vi "LV8_1.vi"() -> ()   [LabVIEW 2011]
uses:
  <vilib>/Analysis/1siggen.llb/Ramp Pattern by Samples.vi
  <vilib>/Analysis/NI_AALBase.lvlib
panel:
  in  "Pole/Zero Location (r/theta) 6":T1={"r"=0.8, "q (in p)"=0.5, "pz"=TRUE, "enable\nenable"=TRUE} {"q (in p)" min=0.0 max=1.0 step=0.1; "r" min=0.0 step=0.1}
  in  "Pole/Zero Location (r/theta) 5":T2={"r"=0.8, "q (in p)"=0.25, "pz"=TRUE, "enable"=TRUE} {"q (in p)" min=0.0 max=1.0 step=0.1; "r" min=0.0 step=0.1}
  in  "Pole/Zero Location (r/theta) 4":T2={"r"=0.6, "q (in p)"=0.0, "pz"=TRUE, "enable"=TRUE} {"q (in p)" min=0.0 max=1.0 step=0.1; "r" min=0.0 step=0.1}
  in  "Pole/Zero Location (r/theta) 3":T2={"r"=1.0, "q (in p)"=1.0, "pz"=FALSE, "enable"=TRUE} {"q (in p)" min=0.0 max=1.0 step=0.1; "r" min=0.0 step=0.1}
  in  "Pole/Zero Location (r/theta) 2":T2={"r"=1.0, "q (in p)"=0.75, "pz"=FALSE, "enable"=TRUE} {"q (in p)" min=0.0 max=1.0 step=0.1; "r" min=0.0 step=0.1}
  out "Y":dbl=1.4000000000000004 min=0.0 max=1.2000000000000002 step=0.1 format="%.3g"
  in  "X":dbl min=0.0 max=3.15 step=0.1 format="%.3g"
  in  "Max FR Mag":dbl=1.4000000000000004 min=1e-05 step=0.1 format="%.3g"
  in  "stop":bool
  out "Gain K":dbl=0.03420443704820256 format="%#.3g"
  out "Pole-Zero Plot":cluster{"Y":dbl[], "Y":dbl[]}[](graph)=[{"Y"=array[4001 elements], "Y"=array[4001 elements]}, {"Y"=[0.6, 0.6, 0.565685424949238, 0.565685424949238, 4.898425415289509e-17, 4.898425415289509e-17], "Y"=[0.0, -0.0, 0.565685424949238, -0.565685424949238, 0.8, -0.8]}, {"Y"=[6.123031769111886e-17, 6.123031769111886e-17, -0.7071067811865475, -0.7071067811865475, -1.0, -1.0], "Y"=[1.0, -1.0, 0.7071067811865476, -0.7071067811865476, 1.2246063538223773e-16, -1.2246063538223773e-16]}, {"Y"=[0.0, 1.0], "Y"=[0.0, 0.0]}]
  out "Magnitude of Frequency Response":cluster{dbl[], "Ramp Pattern":dbl[]}(graph)
  in  "Pole/Zero Location (r/theta) 1":T2={"r"=1.0, "q (in p)"=0.5, "pz"=FALSE, "enable"=TRUE} {"q (in p)" min=0.0 max=1.0 step=0.1; "r" min=0.0 step=0.1}
  # "Filter Design by Pole-Zero Placement"
  # "Vertical Cursor"
  # "+/-"
  # "+/-"
  # "+/-"
  # "+/-"
  # "+/-"
  # "+/-"
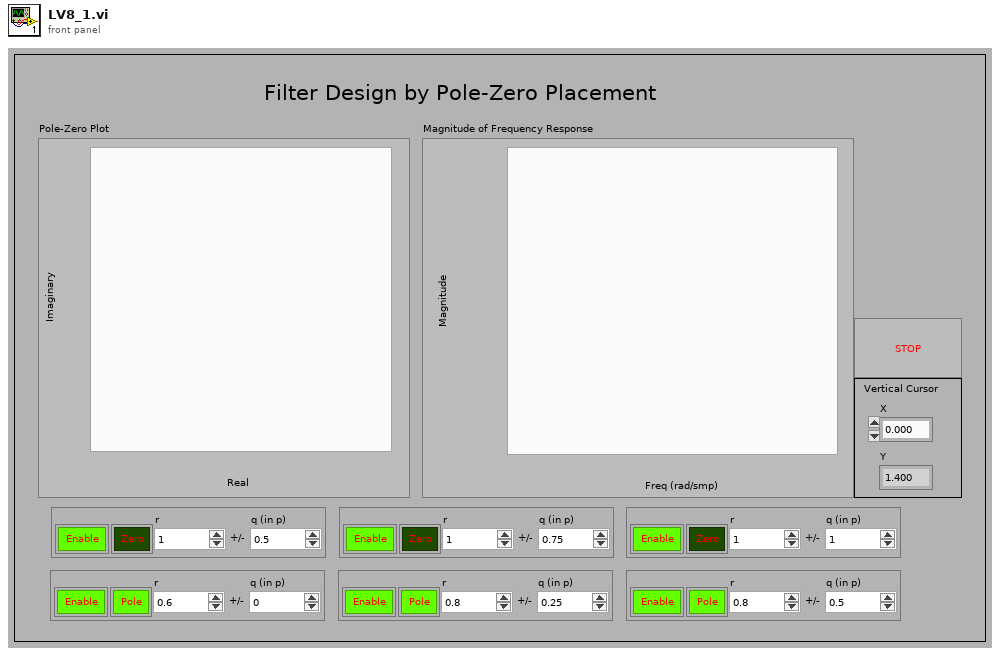
[diagram p1: front panel]
types:
  T1 = cluster{"r":dbl, "q (in p)":dbl, "pz":bool, "enable\nenable":bool}
  T2 = cluster{"r":dbl, "q (in p)":dbl, "pz":bool, "enable":bool}
  T3 = cluster{"r":dbl, "q (in p)":dbl, "pz":bool, "enable\nenable":bool}[]
  T4 = typedef "LVPointDoubleTypeDef.ctl" = cluster{"Cursor X":dbl, "Cursor Y":dbl}
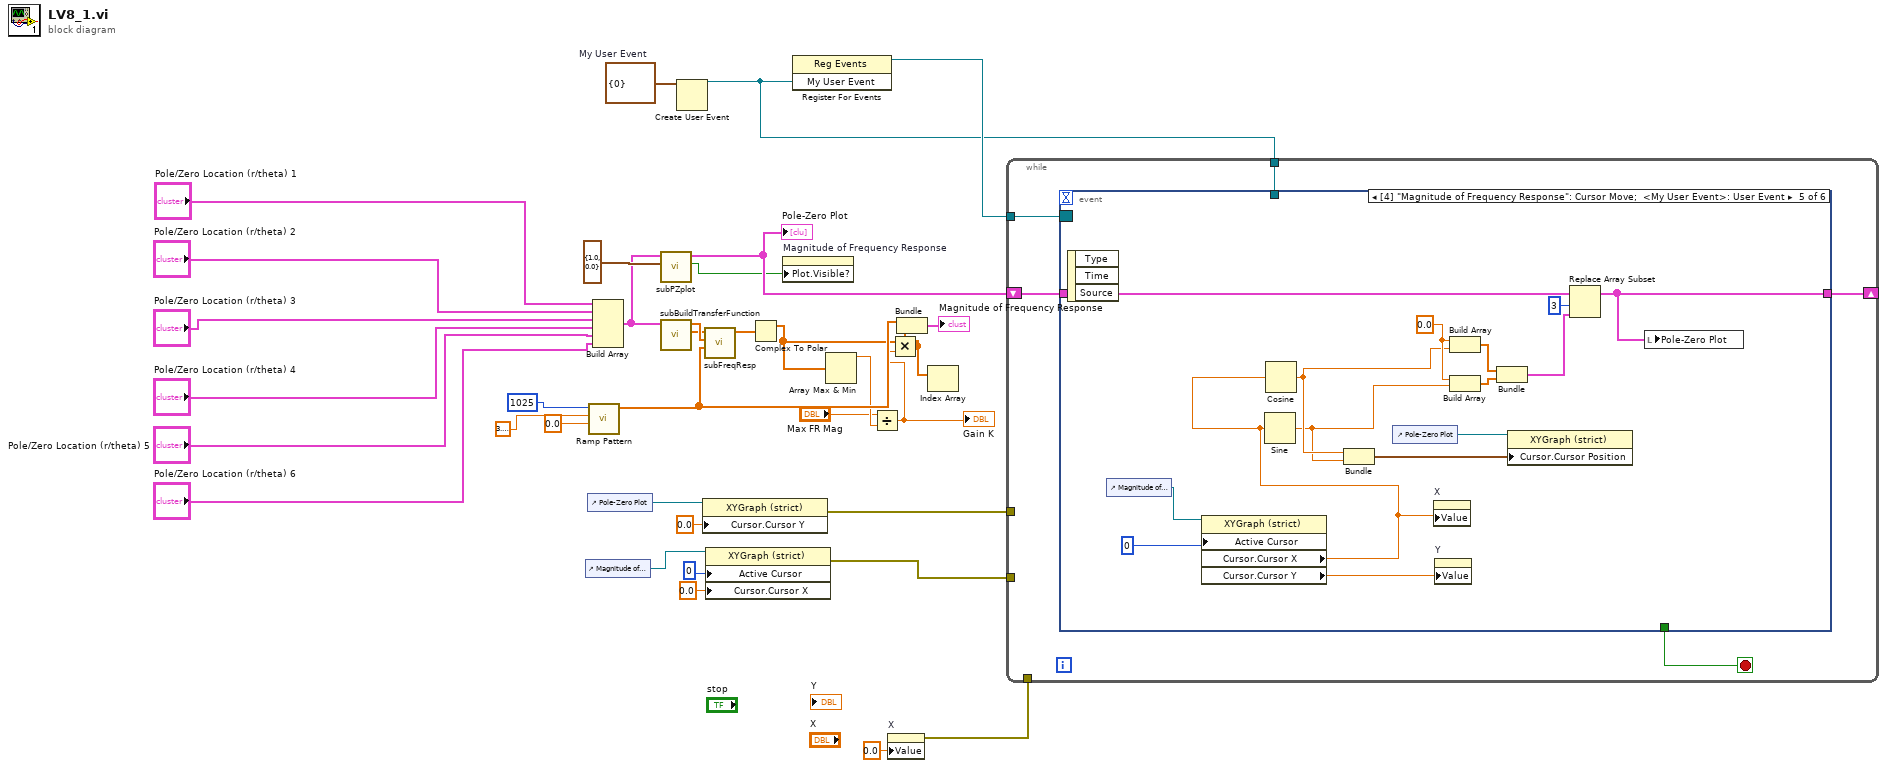
[diagram p0: block diagram]
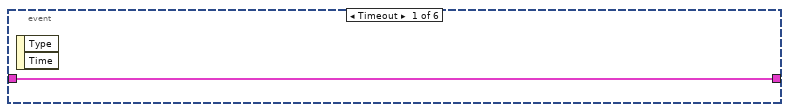
[diagram p2: hidden frame]
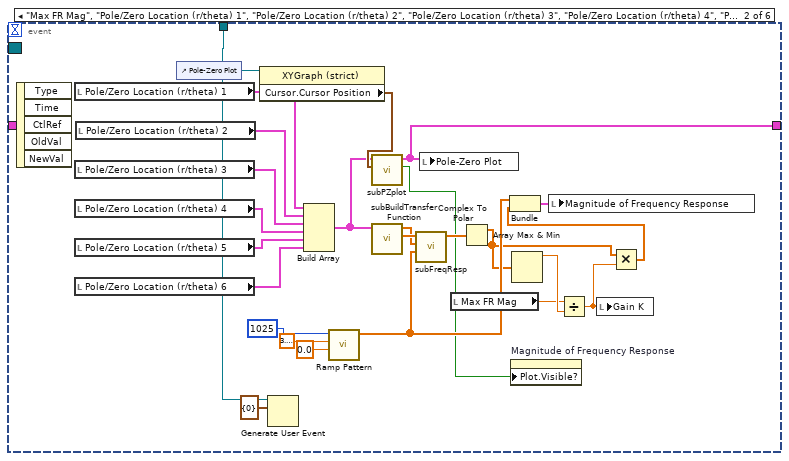
[diagram p3: hidden frame]
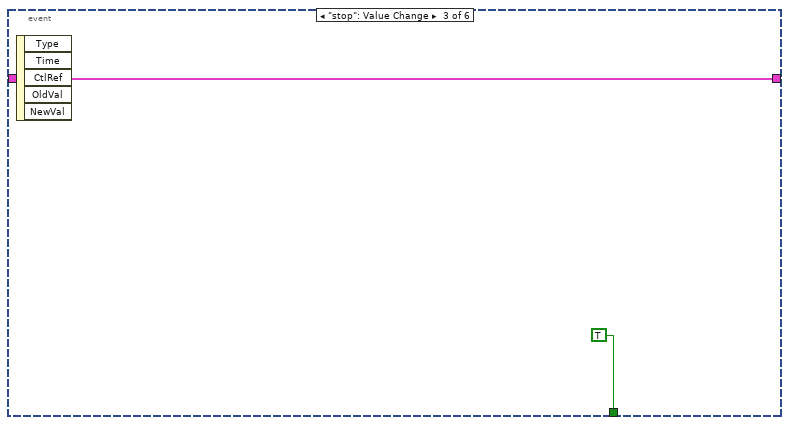
[diagram p4: hidden frame]
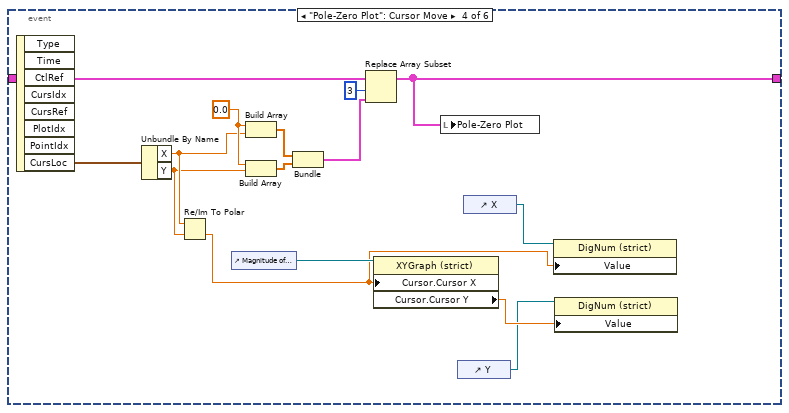
[diagram p5: hidden frame]
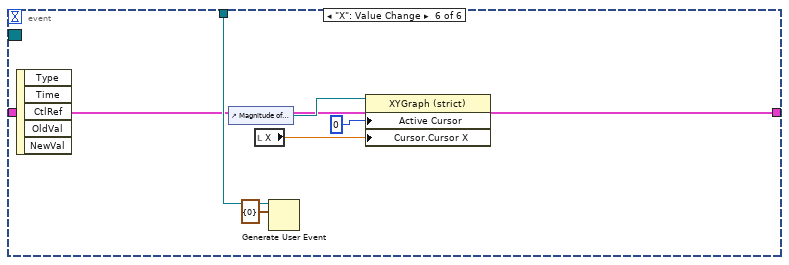
[diagram p6: hidden frame]
diagram:
  w16 = cluster{"dummy":i32} {"dummy"=0}  # My User Event
  n1 = control-ref of="Magnitude of Frequency Response"() -> (w22:refnum<vi>)
  n2 = control-ref of="Pole-Zero Plot"() -> (w25:refnum<vi>)
  n3 = call-poly <vilib>:"Ramp Pattern.vi"("start"=0.0, "end"=3.141592653589793, "samples"=1025) -> ("Ramp Pattern"=w32:dbl[])  [unwired: 7 in, 1 out]
  n4 = Build Array("Pole/Zero Location (r/theta) 1", "Pole/Zero Location (r/theta) 2", "Pole/Zero Location (r/theta) 3", "Pole/Zero Location (r/theta) 4", "Pole/Zero Location (r/theta) 5", "Pole/Zero Location (r/theta) 6") -> (w2:T3)
  n5 = call "subPZplot.vi"("cursor pos"=cluster{"x":dbl, "y":dbl} {"x"=1.0, "y"=0.0}, "PZarray"=w2) -> ("stable？"=w19:bool, "PZplot"=w29:cluster{"Y":dbl[], "Y":dbl[]}[])  [unwired: 8 in]
  "Pole-Zero Plot" <- w29
  n6 = call "subBuildTransferFunction.vi"("PZarray"=w2) -> ("a"=w27:dbl[], "b"=w26:dbl[])  [unwired: 8 in]
  n7 = Create User Event(user event datatype=w16) -> (user event=w15:refnum<user-event>)  [unwired: 1 in, 1 out]
  n8 = property class="XYGraph (strict)"(reference=w25, "Cursor.Cursor Y"=0.0 ("Cursor.Cursor Position:Cursor Y")) -> (error out=w23:errorcluster)  [unwired: 1 in, 1 out]
  n9 = call "subFreqResp.vi"("omega"=w32, "a"=w27, "b"=w26) -> ("Frequency Response"=w35:cdb[])  [unwired: 8 in]
  n10 = property class="XYGraph (strict)"(reference=w22, "Active Cursor"=u32 0, "Cursor.Cursor X"=0.0 ("Cursor.Cursor Position:Cursor Y")) -> (error out=w21:errorcluster)  [unwired: 1 in, 1 out]
  n11 = Complex To Polar(r * e^(i*theta)=w35) -> (r=w13:dbl[])  [unwired: 1 out]
  n12 = property on="Magnitude of Frequency Response" class="XYGraph (strict)"("Plot.Visible?"=w19) -> ()  [unwired: 2 in, 2 out]
  n13 = register-events(w15) -> (reference out=w17:refnum<event-registration>)  [unwired: 2 in, 1 out]
  n14 = Array Max & Min(array=w13) -> (max value=w18:dbl)  [unwired: 3 out]
  n15 = Divide(x="Max FR Mag", y=w18) -> (x/y=w12:dbl)
  "Gain K" <- w12
  n16 = property on="X" class="DigNum (strict)"("Value"=0.0 ("X")) -> (error out=w1:errorcluster)  [unwired: 2 in, 1 out]
  n17 = Multiply(x=w13, y=w12) -> (x*y=w11:dbl[])
  n18 = Bundle("Ramp Pattern"=w32, w11) -> (→"Magnitude of Frequency Response":cluster{"Ramp Pattern":dbl[], dbl[]})  [unwired: 1 in]
  n19 = Index Array(array=w11) -> ()  [unwired: 1 in, 1 out]
  n20 = while {
    shift-right: [w39] -> _
    shift-left: w29 -> [w40]
    tunnel: w23 -> [_]
    tunnel: w21 -> [_]
    tunnel: w17 -> [w37]
    tunnel: w15 -> [w36]
    tunnel: w1 -> [_]
    stop <- w38 stop-if-true
    n21 = event shown="[4] \"Magnitude of Frequency Response\": Cursor Move;  <My User Event>: User Event" {
      selector: w37 -> [_ _ _ _ _ _]
      dyn-events: _ -> [_ _ _ _ _ _]
      timeout: _ -> [_ _ _ _ _ _]
      tunnel: w40 -> [w41 _ w68 w80 w94 w101]
      tunnel: [w41 w58 _ w77 w93 w101] -> w39
      tunnel: [_ _ TRUE _ _ _] -> w38
      tunnel: [_ _ w68 _ _ _] -> _
      tunnel: w36 -> [_ w50 _ _ _ w104]
      event Timeout {
        n22 = event-data() -> ()  [unwired: 1 in, 2 out]
      }
      event "Max FR Mag", "Pole/Zero Location (r/theta) 1", "Pole/Zero Location (r/theta) 2", "Pole/Zero Location (r/theta) 3", "Pole/Zero Location (r/theta) 4", "Pole/Zero Location (r/theta) 5", "Pole/Zero Location (r/theta) 6": Value Change {
        n23 = event-data() -> ()  [unwired: 1 in, 5 out]
        n24 = local read "Pole/Zero Location (r/theta) 1"() -> (w65:T2)
        n25 = local read "Pole/Zero Location (r/theta) 3"() -> (w46:T2)
        n26 = local read "Pole/Zero Location (r/theta) 4"() -> (w45:T2)
        n27 = local read "Pole/Zero Location (r/theta) 5"() -> (w44:T2)
        n28 = local read "Pole/Zero Location (r/theta) 6"() -> (w43:T1)
        n29 = local read "Pole/Zero Location (r/theta) 2"() -> (w47:T2)
        n30 = control-ref of="Pole-Zero Plot"() -> (w67:refnum<vi>)
        n31 = property class="XYGraph (strict)"(reference=w67) -> ("Cursor.Cursor Position"=w57:T4)  [unwired: 1 in, 2 out]
        n32 = Generate User Event(user event=w50, event data cluster=cluster{"dummy":i32} {"dummy"=0} ("event data")) -> ()  [unwired: 1 in, 2 out]
        n33 = Build Array(w65, w47, w46, w45, w44, w43) -> (w42:T3)
        n34 = call-poly <vilib>:"Ramp Pattern.vi"("start"=0.0, "end"=3.141592653589793, "samples"=1025) -> ("Ramp Pattern"=w59:dbl[])  [unwired: 7 in, 1 out]
        n35 = call "subPZplot.vi"("cursor pos"=w57, "PZarray"=w42) -> ("stable？"=w55:bool, "PZplot"=w58:cluster{"Y":dbl[], "Y":dbl[]}[])  [unwired: 8 in]
        n36 = call "subBuildTransferFunction.vi"("PZarray"=w42) -> ("a"=w63:dbl[], "b"=w64:dbl[])  [unwired: 8 in]
        n37 = call "subFreqResp.vi"("omega"=w59, "a"=w63, "b"=w64) -> ("Frequency Response"=w60:cdb[])  [unwired: 8 in]
        n38 = local write "Pole-Zero Plot"(w58) -> ()
        n39 = local read "Max FR Mag"() -> (w48:dbl)
        n40 = Complex To Polar(r * e^(i*theta)=w60) -> (r=w53:dbl[])  [unwired: 1 out]
        n41 = property on="Magnitude of Frequency Response" class="XYGraph (strict)"("Plot.Visible?"=w55) -> ()  [unwired: 2 in, 2 out]
        n42 = Array Max & Min(array=w53) -> (max value=w54:dbl)  [unwired: 3 out]
        n43 = Divide(x=w48, y=w54) -> (x/y=w52:dbl)
        n44 = local write "Gain K"(w52) -> ()
        n45 = Multiply(x=w53, y=w52) -> (x*y=w51:dbl[])
        n46 = Bundle("Ramp Pattern"=w59, w51) -> (w66:cluster{"Ramp Pattern":dbl[], dbl[]})  [unwired: 1 in]
        n47 = local write "Magnitude of Frequency Response"(w66) -> ()
      }
      event "stop": Value Change {
        n48 = event-data() -> ()  [unwired: 1 in, 5 out]
      }
      event "Pole-Zero Plot": Cursor Move {
        w82 = 0.0 ("element")
        n49 = event-data() -> ("CursLoc"=w81:cluster{"X":dbl, "Y":dbl})  [unwired: 1 in, 7 out]
        n50 = Unbundle By Name(w81) -> ("X"=w76:dbl, "Y"=w75:dbl)
        n51 = Re/Im To Polar(2:w75, 3:w76) -> (0:w72:dbl)  [unwired: 1 out]
        n52 = control-ref of="Magnitude of Frequency Response"() -> (w74:refnum<vi>)
        n53 = Build Array(w82, w76) -> (w83:dbl[])
        n54 = Build Array(w82, w75) -> (w84:dbl[])
        n55 = Bundle(w83, w84) -> (w78:cluster{dbl[], dbl[]})  [unwired: 1 in]
        n56 = Replace Array Subset(array=w80, new element=w78, index=3) -> (w77:cluster{"Y":dbl[], "Y":dbl[]}[])
        n57 = property class="XYGraph (strict)"(reference=w74, "Cursor.Cursor X"=w72) -> ("Cursor.Cursor Y"=w71:dbl)  [unwired: 1 in, 2 out]
        n58 = local write "Pole-Zero Plot"(w77) -> ()
        n59 = control-ref of="Y"() -> (w70:refnum<vi>)
        n60 = control-ref of="X"() -> (w73:refnum<vi>)
        n61 = property on="Property Node" class="DigNum (strict)"(reference=w73, "Value"=w72) -> ()  [unwired: 1 in, 2 out]
        n62 = property on="Property Node" class="DigNum (strict)"(reference=w70, "Value"=w71) -> ()  [unwired: 1 in, 2 out]
      }
      event "Magnitude of Frequency Response": Cursor Move; User Event {
        w97 = 0.0 ("element")
        n63 = event-data() -> ()  [unwired: 1 in, 3 out]
        n64 = control-ref of="Magnitude of Frequency Response"() -> (w88:refnum<vi>)
        n65 = property class="XYGraph (strict)"(reference=w88, "Active Cursor"=u32 0) -> ("Cursor.Cursor X"=w87:dbl, "Cursor.Cursor Y"=w86:dbl)  [unwired: 1 in, 2 out]
        n66 = Sine(x=w87) -> (sin(x)=w91:dbl)
        n67 = Cosine(x=w87) -> (cos(x)=w92:dbl)
        n68 = Bundle(w92, w91) -> (w90:cluster{dbl, dbl})  [unwired: 1 in]
        n69 = control-ref of="Pole-Zero Plot"() -> (w89:refnum<vi>)
        n70 = property on="X" class="DigNum (strict)"("Value"=w87) -> ()  [unwired: 2 in, 2 out]
        n71 = property on="Y" class="DigNum (strict)"("Value"=w86) -> ()  [unwired: 2 in, 2 out]
        n72 = Build Array(w97, w92) -> (w98:dbl[])
        n73 = Build Array(w97, w91) -> (w99:dbl[])
        n74 = Bundle(w98, w99) -> (w95:cluster{dbl[], dbl[]})  [unwired: 1 in]
        n75 = property class="XYGraph (strict)"(reference=w89, "Cursor.Cursor Position"=w90) -> ()  [unwired: 1 in, 2 out]
        n76 = Replace Array Subset(array=w94, new element=w95, index=3) -> (w93:cluster{"Y":dbl[], "Y":dbl[]}[])
        n77 = local write "Pole-Zero Plot"(w93) -> ()
      }
      event "X": Value Change {
        n78 = event-data() -> ()  [unwired: 1 in, 5 out]
        n79 = control-ref of="Magnitude of Frequency Response"() -> (w105:refnum<vi>)
        n80 = local read "X"() -> (w102:dbl)
        n81 = Generate User Event(user event=w104, event data cluster=cluster{i32} {0} ("event data")) -> ()  [unwired: 1 in, 2 out]
        n82 = property class="XYGraph (strict)"(reference=w105, "Active Cursor"=0 ("Cursor.Cursor Plot"), "Cursor.Cursor X"=w102) -> ()  [unwired: 1 in, 2 out]
      }
    }
  }
